vi "Clean Up Actor.vi"(8 "error in (no error)":errorcluster, 11 "Mediated Actor in":refnum<class "Mediated Actor.lvclass">) -> (0 "error out":errorcluster, 3 "Mediated Actor out":refnum<class "Mediated Actor.lvclass">)   [LabVIEW 2016, in "Stream Mediator.lvlib" / "Mediated Actor.lvclass"]
doc: "--\nCopyright © 2017 Composed SystemsI All rights reserved.\n\nAuthor: Jon McBee <jon.mcbee@composed.io>\n\nThis library is provided \"AS IS\" ,WITHOUT WARRANTIES OR\nCONDITIONS OF ANY KIND, either express or implied.\n\nComposed Systems -- composed.io\n\nStream 0.0.1.1\nJon McBee - Composed Systems\nCopyright (c) 2017, Composed Systems"
uses:
  <userlib>/Composed Systems/Stream/Mediator/Classes/Mediated Actor/Mediated Actor.lvclass
  <userlib>/Composed Systems/Stream/Mediator/Classes/Mediated Actor/Mediated Actor.lvclass/Mediated Actor.ctl
  <userlib>/Composed Systems/Stream/Mediator/Classes/Message Broker Interface/Message Broker Interface.lvclass
  <userlib>/Composed Systems/Stream/Log/Global Application Log/Global Application Log.lvclass
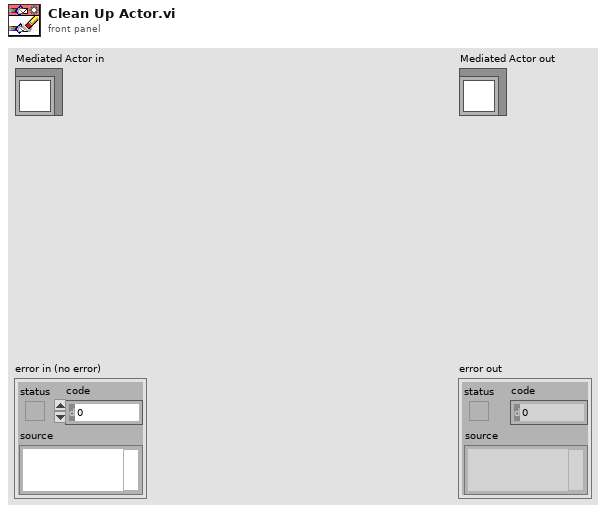
[diagram p1: front panel]
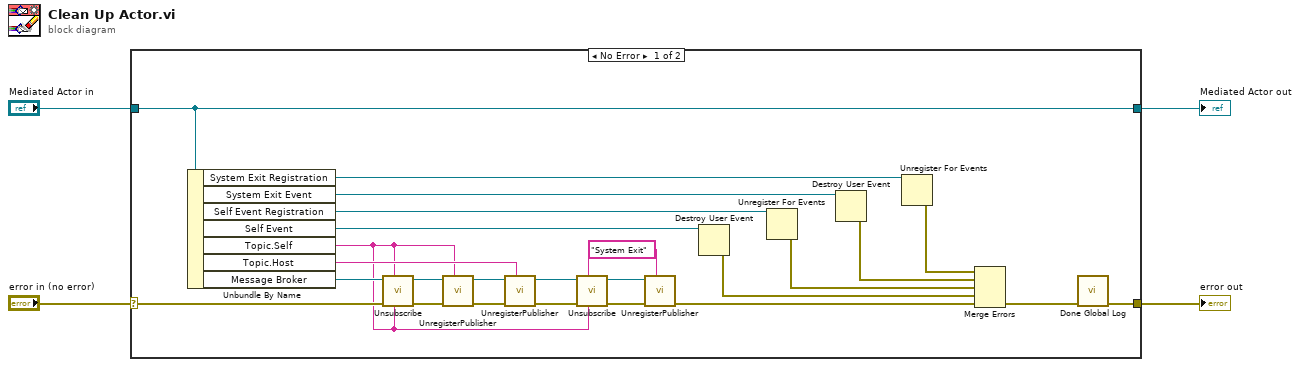
[diagram p0: block diagram]
diagram:
  n1 = case shown="No Error" "error in (no error)" {
    selector: "error in (no error)" -> [w18 w31]
    tunnel: [w16 w31] -> w3
    tunnel: [w29 w30] -> w1
    tunnel: "Mediated Actor in" -> [w29 w30]
    frame No Error {
      w6 = "System Exit" ("Topic Name")
      n2 = Unbundle By Name(w29) -> ("System Exit Registration"=w14:refnum<event-registration>, "System Exit Event"=w15:refnum<user-event>, "Self Event Registration"=w28:refnum<event-registration>, "Self Event"=w27:refnum<user-event>, "Topic.Self"=w5:string, "Topic.Host"=w23:string, "Message Broker"=w26:refnum<class "Message Broker Interface.lvclass">)
      n3 = call-dynamic "Unsubscribe.vi"("Subscriber Name"=w5, "Topic Name"=w5, "error in (no error)"=w18, "Message Broker Interface in"=w26) -> ("error out"=w22:errorcluster, "Message Broker Interface out"=w25:refnum<class "Message Broker Interface.lvclass">)  [unwired: 6 in]
      n4 = call-dynamic "UnregisterPublisher.vi"("Topic Name"=w5, "error in (no error)"=w22, "Message Broker Interface in"=w25) -> ("error out"=w21:errorcluster, "Message Broker Interface out"=w24:refnum<class "Message Broker Interface.lvclass">)  [unwired: 7 in]
      n5 = call-dynamic "UnregisterPublisher.vi"("Topic Name"=w23, "error in (no error)"=w21, "Message Broker Interface in"=w24) -> ("error out"=w11:errorcluster, "Message Broker Interface out"=w8:refnum<class "Message Broker Interface.lvclass">)  [unwired: 7 in]
      n6 = call-dynamic "Unsubscribe.vi"("Subscriber Name"=w5, "Topic Name"=w6, "error in (no error)"=w11, "Message Broker Interface in"=w8) -> ("error out"=w10:errorcluster, "Message Broker Interface out"=w7:refnum<class "Message Broker Interface.lvclass">)  [unwired: 6 in]
      n7 = call-dynamic "UnregisterPublisher.vi"("Topic Name"=w6, "error in (no error)"=w10, "Message Broker Interface in"=w7) -> ("error out"=w9:errorcluster)  [unwired: 7 in, 1 out]
      n8 = Destroy User Event(user event=w27) -> (error out=w19:errorcluster)  [unwired: 1 in]
      n9 = Unregister For Events(event registration refnum=w28) -> (error out=w20:errorcluster)  [unwired: 1 in]
      n10 = Destroy User Event(user event=w15) -> (error out=w12:errorcluster)  [unwired: 1 in]
      n11 = Unregister For Events(event registration refnum=w14) -> (error out=w13:errorcluster)  [unwired: 1 in]
      n12 = Merge Errors(w13, w12, w20, w19, w9) -> (w17:errorcluster)
      n13 = call <userlib>:"Done Global Log.vi"("error in (no error)"=w17) -> ("error out"=w16:errorcluster)  [unwired: 10 in]
    }
    frame Error {
    }
  }
  "error out" <- w3
  "Mediated Actor out" <- w1
